vi "Convert Norm FOV to FOV.vi"(11 "Field of View(norm)":dbl=4.35) -> (0 "error out":errorcluster, 2 "FOV":dbl)   [LabVIEW 2017]
uses:
  Global Variables/General Globals.vi
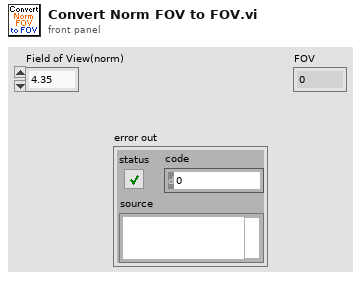
[diagram p1: front panel]
types:
  T1 = typedef "FOV values cluster.ctl" = cluster{"Norm value":sgl, "FOV text":string, "FOV value":i32, "All FOV values":i32[], "All norm FOV values":sgl[], "All FOV value strings":string[], "Strings And Values []":T2}
  T2 = typedef "LVStringsAndValuesArrayTypeDef_SGL.ctl" = cluster{"String":string, "Value":sgl}[]
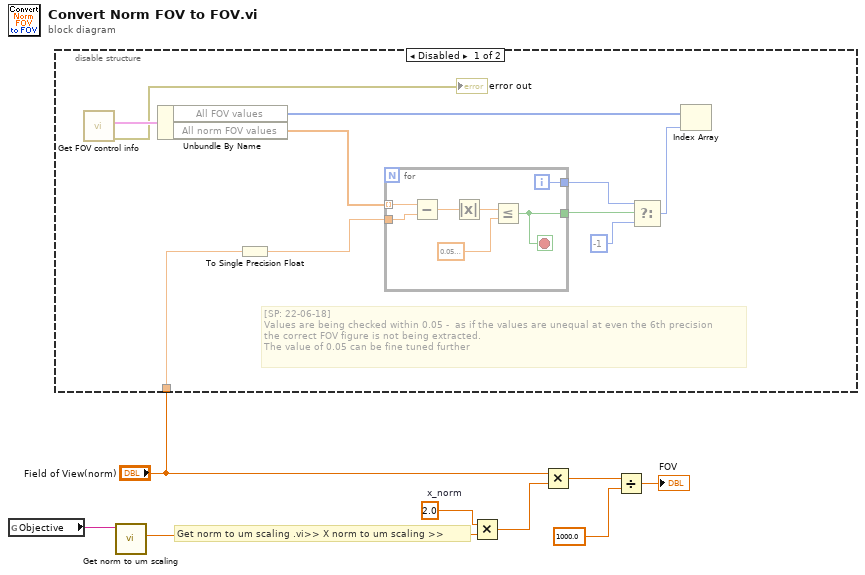
[diagram p0: block diagram]
diagram:
  w6 = 2.0  # x_norm
  # "Get norm to um scaling .vi>> X norm to um scaling >>"
  n1 = global read "General Globals.vi" "Objective"() -> (w5:string)
  n2 = disable-structure shown="Disabled" {
    disable-tunnel: "Field of View(norm)" -> [w9 _]
    frame Disabled {
      # "[SP: 22-06-18]\nValues are being checked within 0.05 -  as if the values are unequal at even the 6th precision\nthe correct FOV figure is not being extracted.\nThe value of 0.05 can be fine tuned further"
      n3 = call "Get FOV control info.vi"() -> ("error out"=→"error out":errorcluster, "FOV values cluster"=w17:T1)  [unwired: 8 in, 2 out]
      n4 = Unbundle By Name(w17) -> ("All FOV values"=w18:i32[], "All norm FOV values"=w10:sgl[])
      n5 = To Single Precision Float(number=w9) -> (single precision float=w15:sgl)
      n6 = for {
        tunnel: w10 -> [w26] mode=indexing
        tunnel: w15 -> [w25]
        tunnel: [w21] -> w13
        tunnel: [w20] -> w14
        i -> [w21]
        stop <- w20 stop-if-true
        n7 = Subtract(x=w26, y=w25) -> (x-y=w24:sgl)
        n8 = Absolute Value(x=w24) -> (abs(x)=w23:sgl)
        n9 = Less Or Equal?(x=w23, y=sgl 0.05) -> (x <= y?=w20:bool)
      }
      n10 = Select(t=w13, s=w14, f=-1) -> (s? t:f=w11:i32)
      n11 = Index Array(array=w18, index=w11) -> (element=w19:i32)
    }
    frame Enabled {
    }
  }
  n12 = call "Get norm to um scaling .vi"("Current Objective"=w5) -> ("X_norm to um_scaling"=w7:dbl)  [unwired: 8 in, 2 out]
  n13 = Multiply(x=w6, y=w7) -> (x*y=w4:dbl)
  n14 = Multiply(x="Field of View(norm)", y=w4) -> (x*y=w3:dbl)
  n15 = Divide(x=w3, y=1000.0) -> (x/y=→"FOV":dbl)
